vi "Open Hardware.vi"(8 "error in (no error)":errorcluster, 11 "Instrument.Oxford1820 in":refnum<class "Instrument.Oxford1820.lvclass">) -> (0 "error out":errorcluster, 3 "Instrument.Oxford1820 out":refnum<class "Instrument.Oxford1820.lvclass">)   [LabVIEW 2019, in "Instrument.Oxford1820.lvclass"]
uses:
  Instrument.Oxford1820.lvclass
  Instrument.Oxford1820.lvclass/Instrument.Oxford1820.ctl
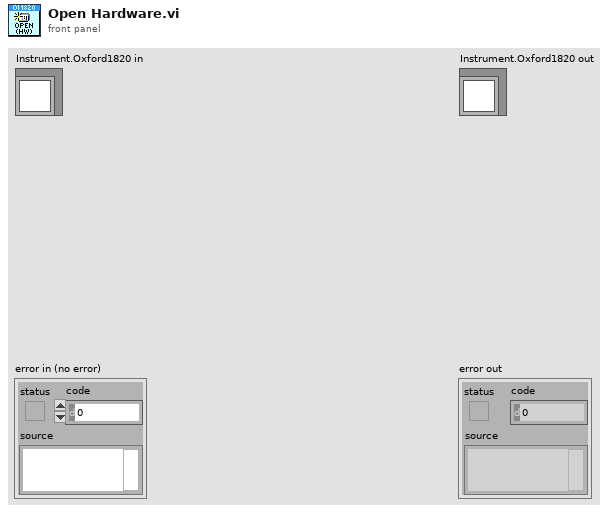
[diagram p1: front panel]
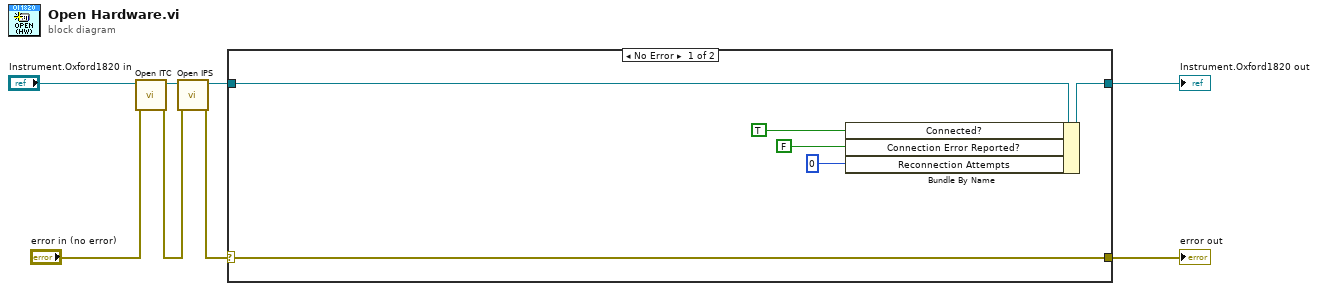
[diagram p0: block diagram]
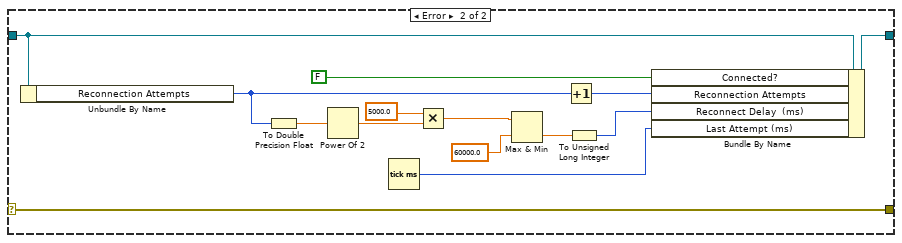
[diagram p2: hidden frame]
diagram:
  n1 = call "Open ITC.vi"("error in (no error)"="error in (no error)", "Instrument.Oxford1820 in"="Instrument.Oxford1820 in") -> ("error out"=w5:errorcluster, "Instrument.Oxford1820 out"=w6:refnum<class "Instrument.Oxford1820.lvclass">)  [unwired: 8 in]
  n2 = call "Open IPS.vi"("error in (no error)"=w5, "Instrument.Oxford1820 in"=w6) -> ("error out"=w3:errorcluster, "Instrument.Oxford1820 out"=w2:refnum<class "Instrument.Oxford1820.lvclass">)  [unwired: 8 in]
  n3 = case shown="No Error" w3 {
    selector: w3 -> [w14 w28]
    tunnel: [w14 w28] -> w4
    tunnel: w2 -> [w10 w25]
    tunnel: [w9 w26] -> w1
    frame No Error {
      n4 = Bundle By Name(cluster=w10, "Connected?"=TRUE ("Connection.Connected?"), "Connection Error Reported?"=FALSE ("Connection.Connection Error Reported?"), "Reconnection Attempts"=u32 0 ("Connection.Reconnection Attempts")) -> (w9:refnum<class "Instrument.Oxford1820.lvclass">)
    }
    frame Error {
      n5 = Unbundle By Name(w25) -> ("Reconnection Attempts"=w17:u32)
      n6 = To Double Precision Float(number=w17) -> (double precision float=w21:dbl)
      n7 = Power Of 2(x=w21) -> (2^x=w18:dbl)
      n8 = Tick Count (ms)() -> (millisecond timer value=w19:u32)
      n9 = Multiply(x=5000.0 ("Connection.Reconnection Attempts"), y=w18) -> (x*y=w20:dbl)
      n10 = Max & Min(x=w20, y=60000.0 ("Connection.Reconnection Attempts")) -> (min(x,y)=w24:dbl)  [unwired: 1 out]
      n11 = Increment(x=w17) -> (x+1=w16:u32)
      n12 = To Unsigned Long Integer(number=w24) -> (unsigned 32bit integer=w15:u32)
      n13 = Bundle By Name(cluster=w25, "Connected?"=FALSE ("Connection.Connected?"), "Reconnection Attempts"=w16, "Reconnect Delay  (ms)"=w15, "Last Attempt (ms)"=w19) -> (w26:refnum<class "Instrument.Oxford1820.lvclass">)
    }
  }
  "error out" <- w4
  "Instrument.Oxford1820 out" <- w1
